vi "Buffer.Get Buffer Size.vi"(11 "Buffer in":refnum<class "Buffer.lvclass">) -> (2 "buffer size":u64, 3 "Buffer out":refnum<class "Buffer.lvclass">)   [LabVIEW 2017, in "DSF Core.lvlib" / "Buffer.lvclass"]
uses:
  Buffer.lvclass
  Buffer.lvclass/Buffer.ctl
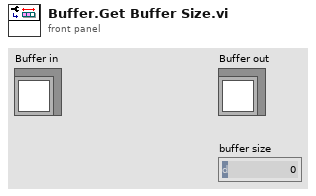
[diagram p1: front panel]
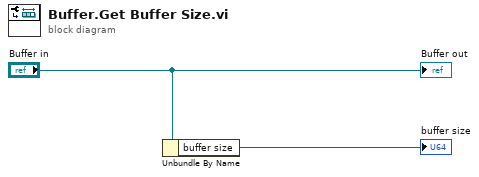
[diagram p0: block diagram]
diagram:
  n1 = Unbundle By Name("Buffer in") -> ("buffer size"=→"buffer size":u64)
  "Buffer out" <- "Buffer in"
